vi "Set Wavelength (SubVI).vi"(2 "error in":errorcluster, 3 "Wavelength (nm)":u32=1064, 4 "VISA Refnum in":refnum<visa-resource-name>) -> (0 "error out":errorcluster, 1 "VISA Refnum out":refnum<visa-resource-name>)   [LabVIEW 2017]
doc: "by Tanguy BOULARD"
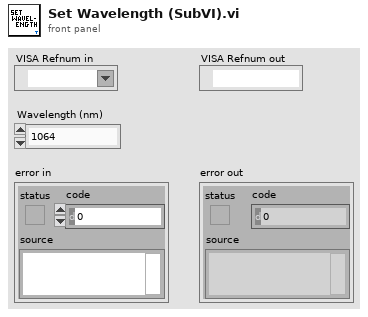
[diagram p1: front panel]
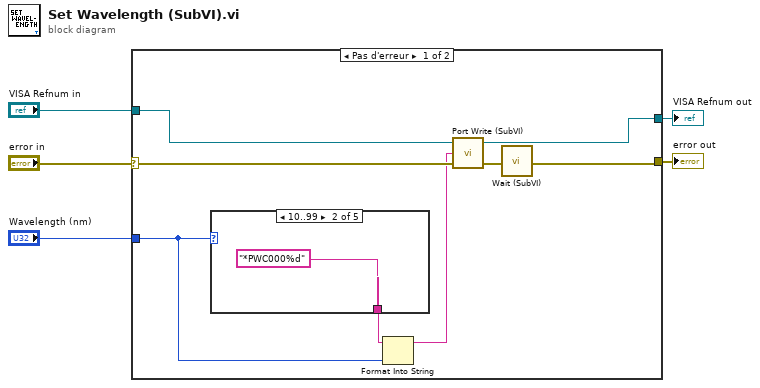
[diagram p0: block diagram]
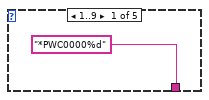
[diagram p2: hidden frame]
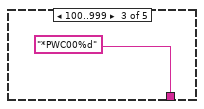
[diagram p3: hidden frame]
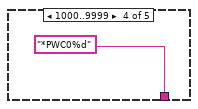
[diagram p4: hidden frame]
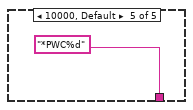
[diagram p5: hidden frame]
diagram:
  n1 = case shown="Pas d'erreur" "error in" {
    selector: "error in" -> [w13 w20]
    tunnel: [w8 w20] -> w2
    tunnel: "VISA Refnum in" -> [w6 w19]
    tunnel: [w9 w19] -> w4
    tunnel: "Wavelength (nm)" -> [w11 _]
    frame No Error {
      n2 = case shown="10..99" w11 {
        tunnel: ["*PWC0000%d" ("format string") "*PWC000%d" ("format string") "*PWC00%d" ("format string") "*PWC0%d" ("format string") "*PWC%d" ("format string")] -> w12
        frame 1..9 {
        }
        frame 10..99 {
        }
        frame 100..999 {
        }
        frame 1000..9999 {
        }
        frame 10000, Default {
        }
      }
      n3 = Format Into String(format string=w12, w11) -> (resulting string=w7:string)  [unwired: 2 in, 1 out]
      n4 = call "Port Write (SubVI).vi"("error in"=w13, "write buffer"=w7, "VISA Refnum in"=w6) -> ("error out"=w10:errorcluster, "VISA Refnum out"=w9:refnum<visa-resource-name>)  [unwired: 1 in]
      n5 = call "Wait (SubVI).vi"("error in"=w10) -> ("error out"=w8:errorcluster)  [unwired: 26 in]
    }
    frame Error {
    }
  }
  "error out" <- w2
  "VISA Refnum out" <- w4
